vi "Return space.vi"(0 "System no.":i32=1 min=1 max=4 step=1, 1 "With space?":bool) -> (14 "String out":string, 15 "Space returned?":bool)   [LabVIEW 2026]
doc: "This VI returns a space character in String out if With space? is TRUE or GCS syntax version is higher than 1.0."
uses:
  Communication/Syntax.ctl
  Communication/Global1.vi
panel:
  # "This VI returns a space character\nin \"String out\" if \"With space?\" is \nTRUE or GCS syntax version is \nhigher than 1.0."
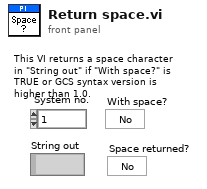
[diagram p1: front panel]
types:
  T1 = typedef "Syntax.ctl" = enum16{"GCS 1.0", "GCS 2.0", "GCS 3.0"}
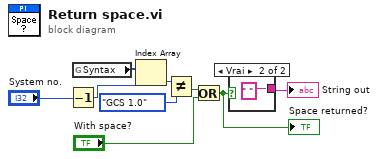
[diagram p0: block diagram]
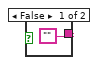
[diagram p2: hidden frame]
diagram:
  n1 = Decrement(x="System no.") -> (x-1=w5:i32)
  n2 = global read "Global1.vi" "Syntax"() -> (w4:T1[])
  n3 = Index Array(array=w4, index=w5) -> (element=w7:T1)
  n4 = Not Equal?(x=w7, y=Syntax."GCS 1.0" ("Syntax")) -> (x != y?=w8:bool)
  n5 = Or(x=w8, y="With space?") -> (x .or. y?=w2:bool)
  "Space returned?" <- w2
  n6 = case shown="Vrai" w2 {
    tunnel: ["" " "] -> w6
    frame False {
    }
    frame True {
    }
  }
  "String out" <- w6
